vi "Write Protocol.vi"(8 "error in (no error)":errorcluster, 10 "Protocol":T1=enum."TCPIP", 11 "Listener in":refnum<class "Listener.lvclass">) -> (0 "error out":errorcluster, 3 "Listener out":refnum<class "Listener.lvclass">)   [LabVIEW 2019, in "Listener.lvclass"]
uses:
  Listener.lvclass
  ListenerClassControls/Protocol Ctl.ctl
  Listener.lvclass/Listener.ctl
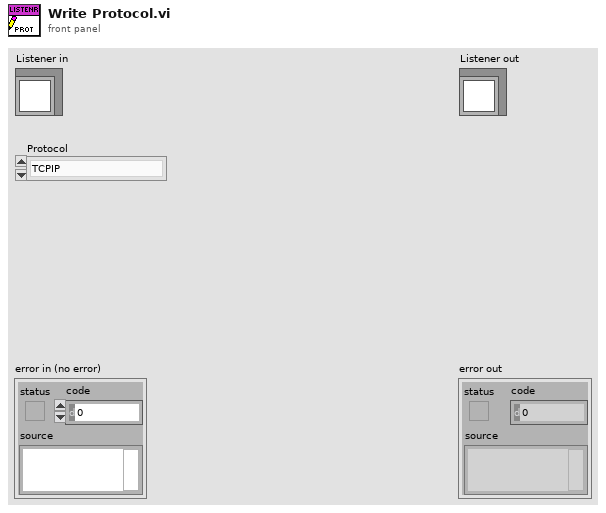
[diagram p1: front panel]
types:
  T1 = typedef "Listener.lvclass/Protocol Ctl.ctl" = enum16{"RS-XXX", "VISA", "TCPIP", "UDP", "GPIB ConvBox"}
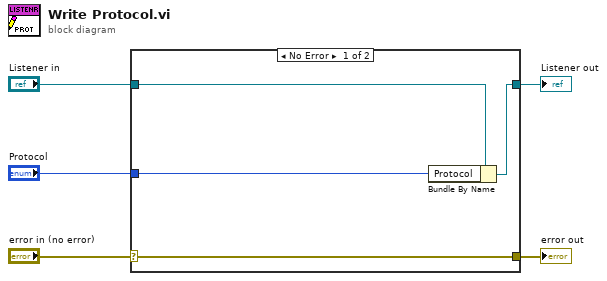
[diagram p0: block diagram]
diagram:
  n1 = case shown="No Error" "error in (no error)" {
    selector: "error in (no error)" -> [w9 w10]
    tunnel: [w9 w10] -> w4
    tunnel: [w7 w11] -> w2
    tunnel: "Listener in" -> [w8 w11]
    tunnel: "Protocol" -> [w6 _]
    frame No Error {
      n2 = Bundle By Name(cluster=w8, "Protocol"=w6) -> (w7:refnum<class "Listener.lvclass">)
    }
    frame Error {
    }
  }
  "error out" <- w4
  "Listener out" <- w2
